vi "Read_Light_Tester.vi"   [LabVIEW 2016]
uses:
  <vilib>/NXT/Dual Mode Library/Display/clearDisplay.vi
  <vilib>/NXT/Dual Mode Library/Display/drawText.vi
  <vilib>/NXT/Dual Mode Library/Display/drawNumber_float.vi
  <vilib>/NXT/Dual Mode Library/Waits/Wait_Num.vi
types:
  T1 = typedef "LVHSConnector.ctl" = refnum<class "BrickReference.lvclass">
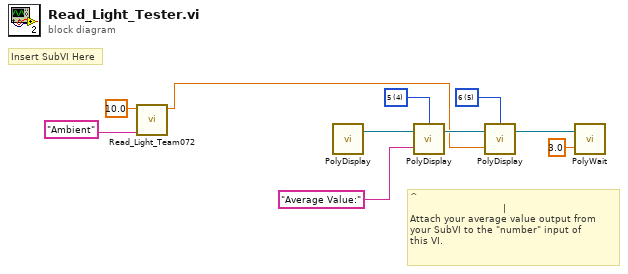
[diagram p0: block diagram]
diagram:
  w9 = i16 5 items=["1", "2", "3", "4", "5", "6", "7", "8", "9", "10", "11", "12"] ("Line")
  w10 = i16 4 items=["1", "2", "3", "4", "5", "6", "7", "8", "9", "10", "11", "12"] ("Line")
  # "^\n                               |\nAttach your average value output from \nyour SubVI to the \"number\" input of\nthis VI."
  # "Insert SubVI Here"
  n1 = call "Read_Light_Team072.vi"("Color Sensing Mode"="Ambient", "Number of Measurements to Take"=10.0) -> ("Average Measurement Value"=w3:dbl)  [unwired: 9 in]
  n2 = call-poly <vilib>:"PolyDisplay.vi"() -> ("NXT/EV3"=w8:T1)  [unwired: 4 in]
  n3 = call-poly <vilib>:"PolyDisplay.vi"("Text"="Average Value:", "NXT/EV3"=w8, "Line"=w10) -> ("NXT/EV3"=w7:T1)  [unwired: 1 in]
  n4 = call-poly <vilib>:"PolyDisplay.vi"("number"=w3, "NXT/EV3"=w7, "Line"=w9) -> ("NXT/EV3"=w6:T1)  [unwired: 1 in]
  n5 = call-poly <vilib>:"PolyWait.vi"("Time (1 sec)"=sgl 3.0, "NXT/EV3"=w6) -> ()  [unwired: 2 in, 1 out]
